vi "Query firmware version.vi"() -> ()   [LabVIEW 2016, in "Drivers.lvlib" / "Agilis.lvlib"]
uses:
  Agilis.lvlib
panel:
  out "Firmware Version":string
  in  "Port":refnum<visa-resource-name>
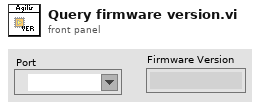
[diagram p1: front panel]
types:
  T1 = typedef "AgilisCmdLib Refnum.ctl" = refnum<k24>
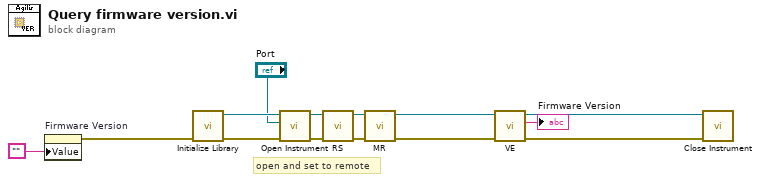
[diagram p0: block diagram]
diagram:
  # "open and set to remote"
  n1 = property on="Firmware Version" class="Str"("Value"="") -> (error out=w6:errorcluster)  [unwired: 2 in, 1 out]
  n2 = call "Initialize Library.vi"("error in (no error)"=w6) -> ("error out"=w13:errorcluster, "Agilis out"=w14:T1)  [unwired: 9 in]
  n3 = call "Open Instrument.vi"("error in (no error)"=w13, "Device Key"="Port", "Agilis in"=w14) -> ("error out"=w3:errorcluster, "Agilis out"=w4:T1)  [unwired: 7 in]
  n4 = call "RS.vi"("error in (no error)"=w3, "Agilis in"=w4) -> ("error out"=w2:errorcluster, "Agilis out"=w1:T1)  [unwired: 8 in]
  n5 = call "MR.vi"("error in (no error)"=w2, "Agilis in"=w1) -> ("error out"=w10:errorcluster, "Agilis out"=w11:T1)  [unwired: 8 in]
  n6 = call "VE.vi"("error in (no error)"=w10, "Agilis in"=w11) -> ("error out"=w8:errorcluster, "Firmware Version"=→"Firmware Version":string, "Agilis out"=w9:T1)  [unwired: 7 in]
  n7 = call "Close Instrument.vi"("error in (no error)"=w8, "Agilis in"=w9) -> ()  [unwired: 9 in, 1 out]
